vi "Day03-2.vi"() -> ()   [LabVIEW 2021]
panel:
  out "Life Support":u32
  out "CO2 Scrubber":u32
  out "Oxygen":u32
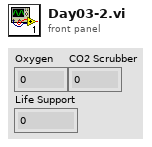
[diagram p1: front panel]
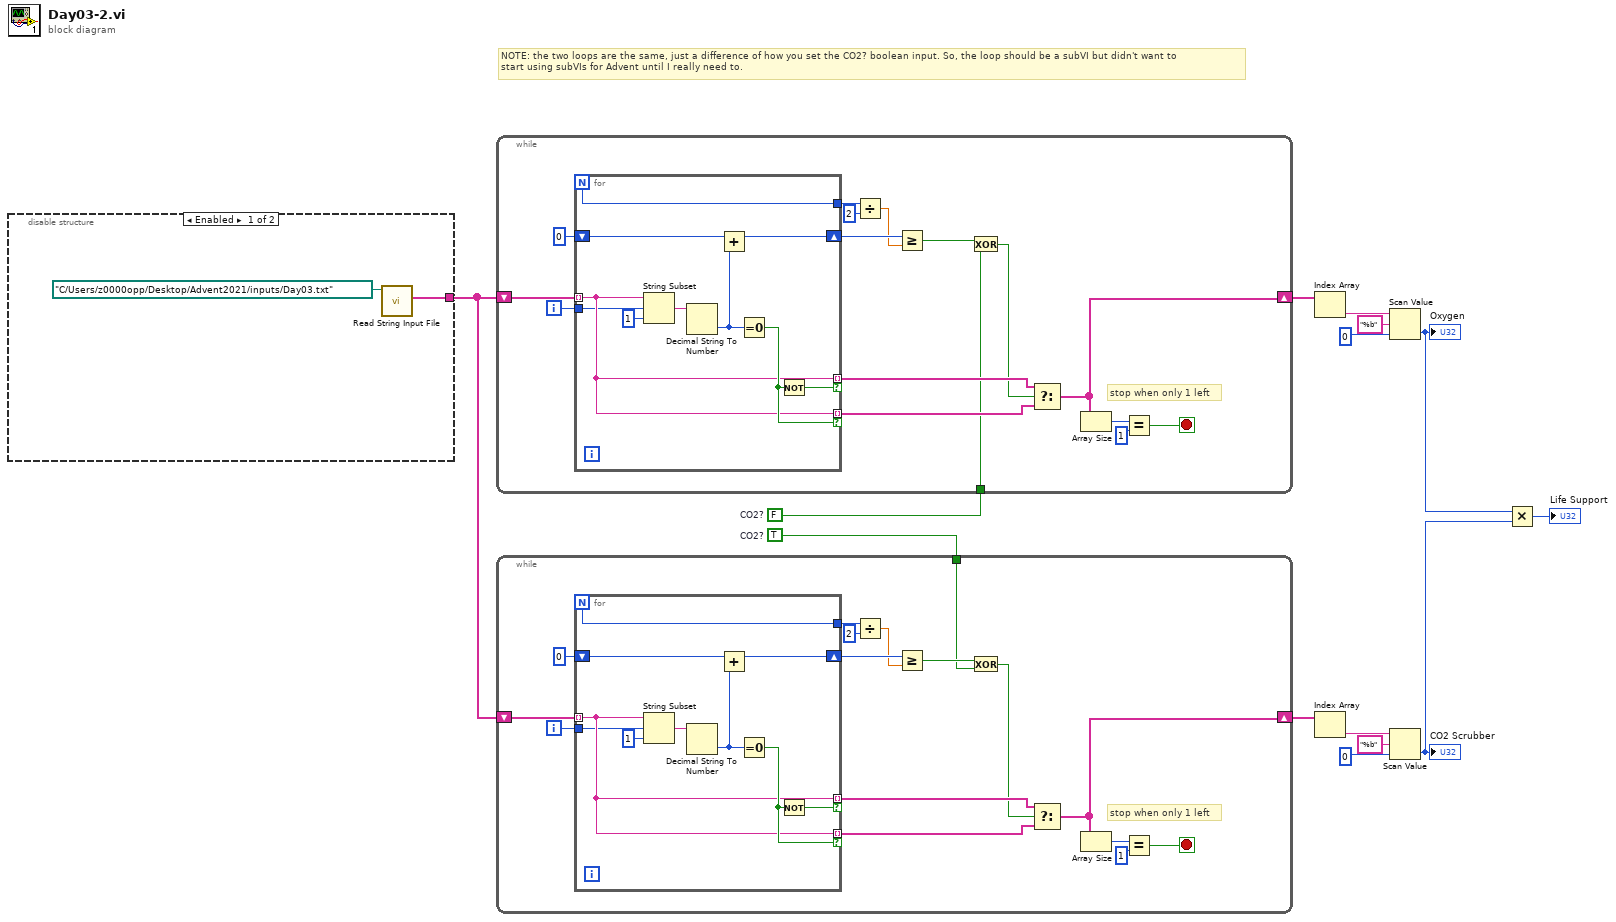
[diagram p0: block diagram]
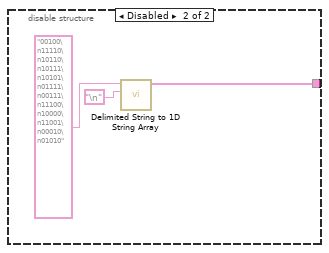
[diagram p2: hidden frame]
diagram:
  w1 = TRUE  # CO2?
  w6 = FALSE  # CO2?
  # "NOTE: the two loops are the same, just a difference of how you set the CO2? boolean input. So, the loop should be a subVI but didn't want to \nstart using subVIs for Advent until I really need to."
  n1 = disable-structure shown="Enabled" {
    disable-tunnel: [w15 w17] -> w5
    frame Enabled {
      n2 = call "Read String Input File.vi"("file path (dialog if empty)"=path "C:/Users/z0000opp/Desktop/Advent2021/inputs/Day03.txt") -> ("input values"=w15:string[])  [unwired: 10 in]
    }
    frame Disabled {
      n3 = call <vilib>:"Delimited String to 1D String Array.vi"("delimiter"="\n", "delimited string"="00100\n11110\n10110\n10111\n10101\n01111\n00111\n11100\n10000\n11001\n00010\n01010") -> ("string array"=w17:string[])  [unwired: 9 in]
    }
  }
  n4 = while {
    shift-right: [w26] -> w13
    shift-left: w5 -> [w35]
    tunnel: w6 -> [w20]
    i -> [w23]
    stop <- w27 stop-if-true
    # "stop when only 1 left"
    n5 = for {
      N -> [w43]
      tunnel: w35 -> [w40] mode=indexing
      shift-right: [w44] -> w33
      shift-left: 0 -> [w45]
      tunnel: [w43] -> w32
      tunnel: [w40] -> w25 mode=indexing if=w42
      tunnel: [w40] -> w24 mode=indexing if=w41
      tunnel: w23 -> [w39]
      n6 = String Subset(string=w40, offset (0)=w39, length (rest)=1 ("length (rest)")) -> (substring=w37:string)
      n7 = Decimal String To Number(string=w37) -> (number=w36:i32)  [unwired: 2 in, 1 out]
      n8 = Add(x=w45, y=w36) -> (x+y=w44:i32)
      n9 = Equal To 0?(x=w36) -> (x = 0?=w41:bool)
      n10 = Not(x=w41) -> (.not. x?=w42:bool)
    }
    n11 = Divide(x=w32, y=2) -> (x/y=w30:dbl)
    n12 = Greater Or Equal?(x=w33, y=w30) -> (x >= y?=w22:bool)
    n13 = Exclusive Or(1:w20, 2:w22) -> (0:w21:bool)
    n14 = Select(t=w25, s=w21, f=w24) -> (s? t:f=w26:string[])
    n15 = Array Size(array=w26) -> (size(s)=w29:i32)
    n16 = Equal?(x=w29, y=1) -> (x = y?=w27:bool)
  }
  n17 = while {
    shift-right: [w52] -> w4
    shift-left: w5 -> [w61]
    tunnel: w1 -> [w46]
    i -> [w49]
    stop <- w53 stop-if-true
    # "stop when only 1 left"
    n18 = for {
      N -> [w69]
      tunnel: w61 -> [w66] mode=indexing
      shift-right: [w70] -> w59
      shift-left: 0 -> [w71]
      tunnel: [w69] -> w58
      tunnel: [w66] -> w51 mode=indexing if=w68
      tunnel: [w66] -> w50 mode=indexing if=w67
      tunnel: w49 -> [w65]
      n19 = String Subset(string=w66, offset (0)=w65, length (rest)=1 ("length (rest)")) -> (substring=w63:string)
      n20 = Decimal String To Number(string=w63) -> (number=w62:i32)  [unwired: 2 in, 1 out]
      n21 = Add(x=w71, y=w62) -> (x+y=w70:i32)
      n22 = Equal To 0?(x=w62) -> (x = 0?=w67:bool)
      n23 = Not(x=w67) -> (.not. x?=w68:bool)
    }
    n24 = Divide(x=w58, y=2) -> (x/y=w56:dbl)
    n25 = Greater Or Equal?(x=w59, y=w56) -> (x >= y?=w48:bool)
    n26 = Exclusive Or(1:w46, 2:w48) -> (0:w47:bool)
    n27 = Select(t=w51, s=w47, f=w50) -> (s? t:f=w52:string[])
    n28 = Array Size(array=w52) -> (size(s)=w55:i32)
    n29 = Equal?(x=w55, y=1) -> (x = y?=w53:bool)
  }
  n30 = Index Array(array=w13) -> (element=w12:string)  [unwired: 1 in]
  n31 = Index Array(array=w4) -> (element=w9:string)  [unwired: 1 in]
  n32 = Scan Value(string=w12, format string="%b", default (0 dbl)=u32 0) -> (value=w2:u32)  [unwired: 1 out]
  "Oxygen" <- w2
  n33 = Scan Value(string=w9, format string="%b", default (0 dbl)=u32 0) -> (value=w3:u32)  [unwired: 1 out]
  "CO2 Scrubber" <- w3
  n34 = Multiply(x=w2, y=w3) -> (x*y=→"Life Support":u32)
